vi "low_pass_filter_3rd.vi"(7 "Input":dbl format="%.2f", 13 "Corner period":dbl(slide)=10.237739663395852 scale=1.0..1000.0) -> (8 "Output":dbl format="%.2f")   [LabVIEW 2016]
doc: "Use this VI to filter a signal using 3rd order low pass filter. The difference equation is \n[y(j)-3*y(j-1)+3*y(j-2)-y(j-3)] + 2*b*[y(j)-2*y(j-1)+y(j-2)] + 2*(b^2)*[y(j)-y(j-1)] + (b^3)*y(j) = (b^3)*x(j).\n\nInputs:\nInput,\nCorner period.\nOutputs:\nOutput.\n\nMuhannad Alghamdi\nCSUSB Physics 350"
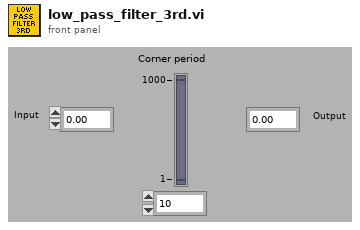
[diagram p1: front panel]
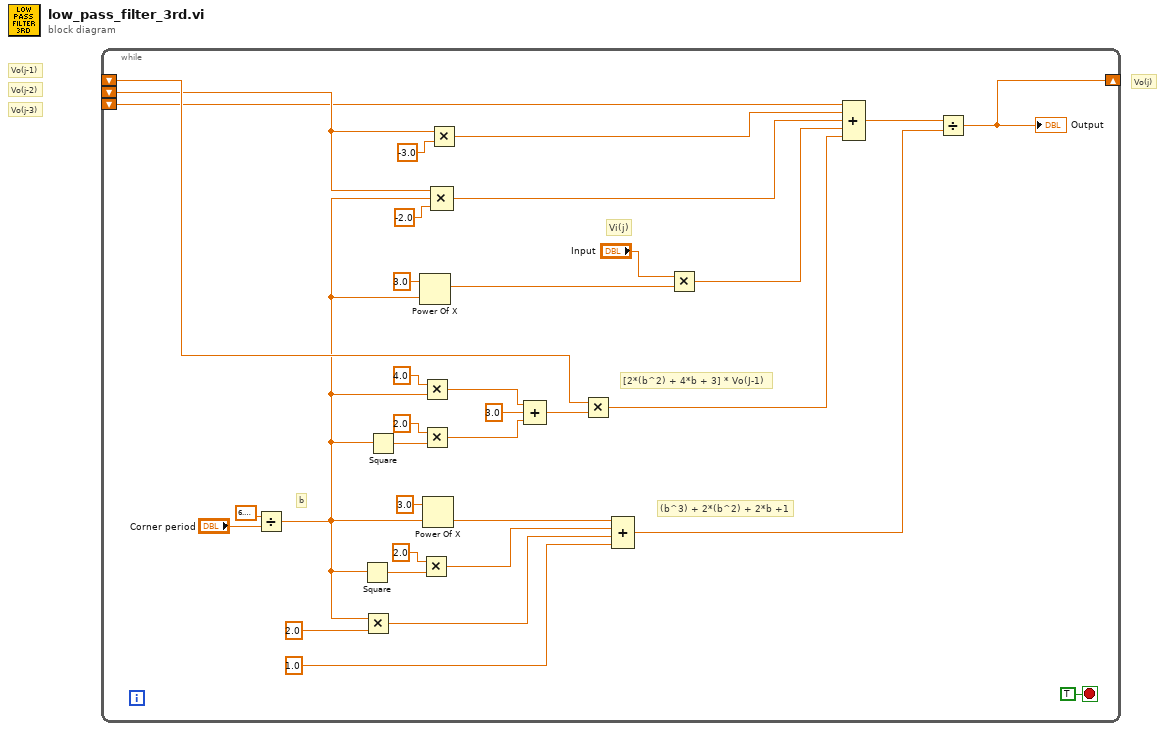
[diagram p0: block diagram]
diagram:
  # "Vo(j-3)"
  # "Vo(j-1)"
  # "Vo(j-2)"
  # "Vo(j)"
  n1 = while {
    shift-left: _ -> [w13]
    shift-right: [w30] -> _
    shift-left: _ -> [w11]
    shift-left: _ -> [w7]
    stop <- TRUE stop-if-true
    # "[2*(b^2) + 4*b + 3] * Vo(J-1)"
    # "Vi(j)"
    # "(b^3) + 2*(b^2) + 2*b +1"
    # "b"
    n2 = Divide(x=6.283185307179586, y="Corner period") -> (x/y=w2:dbl)
    n3 = Square(x=w2) -> (x^2=w19:dbl)
    n4 = Multiply(x=w2, y=2.0 ("x")) -> (x*y=w28:dbl)
    n5 = Square(x=w2) -> (x^2=w25:dbl)
    n6 = Power Of X(1:w2, 2:3.0 ("y")) -> (0:w3:dbl)
    n7 = Multiply(x=2.0, y=w19) -> (x*y=w17:dbl)
    n8 = Multiply(x=4.0, y=w2) -> (x*y=w23:dbl)
    n9 = Multiply(x=2.0, y=w25) -> (x*y=w22:dbl)
    n10 = Power Of X(1:w2, 2:3.0 ("y")) -> (0:w16:dbl)
    n11 = Multiply(x=w11, y=-3.0) -> (x*y=w8:dbl)
    n12 = Compound Arithmetic op=MULTIPLY(w11, w2, -2.0 ("value")) -> (w9:dbl)
    n13 = Compound Arithmetic op=ADD(w23, 3.0 ("value"), w22) -> (w14:dbl)
    n14 = Multiply(x=w13, y=w14) -> (x*y=w4:dbl)
    n15 = Compound Arithmetic op=ADD(w16, w17, w28, 1.0 ("value")) -> (w29:dbl)
    n16 = Multiply(x="Input", y=w3) -> (x*y=w5:dbl)
    n17 = Compound Arithmetic op=ADD(w7, w8, w9, w5, w4) -> (w31:dbl)
    n18 = Divide(x=w31, y=w29) -> (x/y=w30:dbl)
    "Output" <- w30
  }
